vi "Test Process Multiple Parallell Processes.vi"(8 "error in (no error)":errorcluster, 11 "Rig Test In":refnum<class "Process Dev Test.lvclass">) -> (0 "error out":errorcluster, 3 "Rig Test Out":refnum<class "Process Dev Test.lvclass">)   [LabVIEW 2020, in "Process Dev Test.lvclass"]
uses:
  Process Dev Test.lvclass
  C:/Program Files (x86)/National Instruments/LabVIEW 2020/vi.lib/Astemes/LUnit/Test Case.lvclass
  source/Framework Test Suite/Mock Error Handler/Mock Error Handler.lvclass
  C:/Git/triarc-framework/source/Framework/Error Handler Interface/Error Handler Interface.lvclass
  source/Framework/Process/Process.lvclass
  source/Framework/Process/Process.lvclass/Process.ctl
  <vilib>/Astemes/LUnit/Test Case.lvclass/Test Case.ctl
  <vilib>/Astemes/LUnit/LUnit Assertion Result.lvclass/LUnit Assertion Result.ctl
  <vilib>/Astemes/LUnit/LUnit Test Case Result.lvclass/LUnit Test Case Result.ctl
  <vilib>/Astemes/LUnit/LUnit Method Result.lvclass/LUnit Method Result.ctl
  source/Framework/Process/Protected/Messaging/Enqueue Message.vi
  source/Framework/Process/Public/Lifecycle/Get Lifecycle State.vi
  source/Framework/Process/Private/SubVIs/Wait for finish.vi
  source/Framework/Process/Private/SubVIs/Set Lifecycle State.vi
  <vilib>/Astemes/LUnit/Set Assertion Type.vi
  <vilib>/Astemes/LUnit/Palette/Pass.vi
  <vilib>/Astemes/LUnit/Palette/Fail.vi
  source/Framework/Process/Private/SubVIs/Handle Debug Data.vi
  <vilib>/Utility/error.llb/Clear Errors.vi
  <vilib>/Astemes/LUnit/LUnit Write Assertion Type.vi
  <vilib>/Astemes/LUnit/Add test result.vi
  <vilib>/Astemes/LUnit/LUnit Write Passed.vi
  <vilib>/Astemes/LUnit/LUnit Write Message.vi
  <vilib>/Astemes/LUnit/LUnit Write Description.vi
  source/Framework/Logging/Log Debug.vi
  <vilib>/AdvancedString/1D String Array to Delimited String.vi
  <vilib>/Utility/High Resolution Relative Seconds.vi
  <vilib>/Astemes/LUnit/LUnit Record Assertion Result.vi
  <vilib>/Astemes/LUnit/LUnit Aggregate Assertion Results.vi
  <vilib>/Astemes/LUnit/Assertion Result/LUnit Read Status.vi
  <vilib>/Astemes/LUnit/LUnit Read Message.vi
  <vilib>/Astemes/LUnit/LUnit Read Description.vi
  <vilib>/Astemes/LUnit/Method Result/LUnit Merge Status.vi
  <vilib>/Astemes/LUnit/LUnit Concatenate result strings.vi
  <vilib>/Utility/error.llb/Error Cluster From Error Code.vi
  source/Framework/Process/Public/Read Name.vi
  <vilib>/Astemes/LUnit/LUnit Assertion Result.lvclass
  <vilib>/Astemes/LUnit/Test Case.lvclass
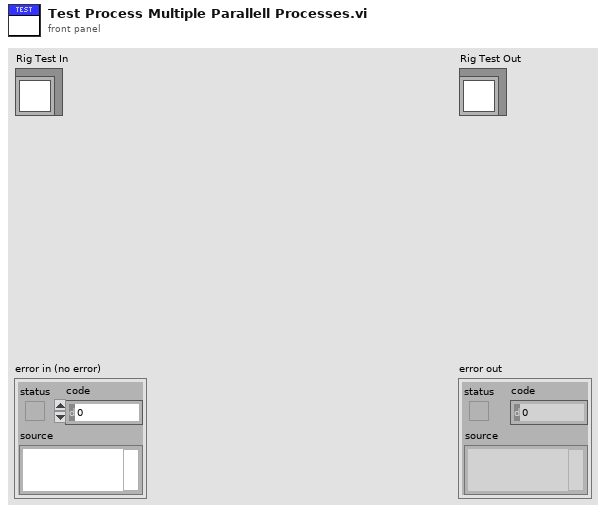
[diagram p1: front panel]
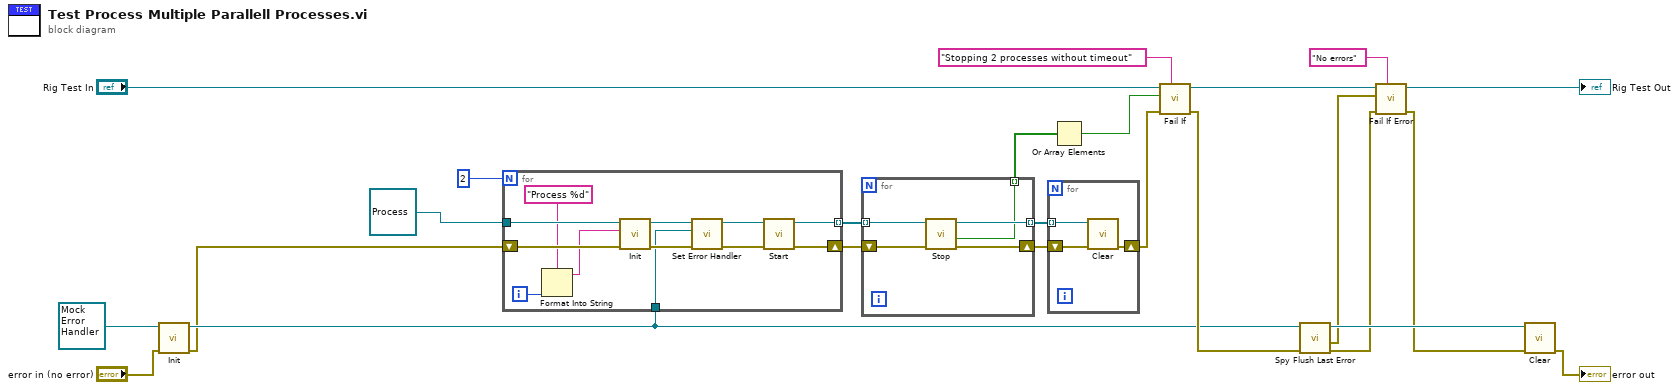
[diagram p0: block diagram]
diagram:
  n1 = call-dynamic "Init.vi"("error in (no error)"="error in (no error)", "Mock Error Handler In"=refnum<class "Mock Error Handler.lvclass"> refnum ("Mock Error Handler.lvclass")) -> ("error out"=w3:errorcluster, "Mock Error Handler Out"=w6:refnum<class "Mock Error Handler.lvclass">)  [unwired: 8 in]
  n2 = for {
    N: 2 -> [_]
    tunnel: [w36] -> w23 mode=indexing
    tunnel: refnum<class "Process.lvclass"> refnum ("Process.lvclass") -> [w33]
    shift-right: [w35] -> w22
    shift-left: w3 -> [w34]
    tunnel: w6 -> [w28]
    i -> [w26]
    n3 = Format Into String(format string="Process %d", w26) -> (resulting string=w25:string)  [unwired: 2 in, 1 out]
    n4 = call-dynamic "Init.vi"("error in (no error)"=w34, "Name"=w25, "Process In"=w33) -> ("error out"=w30:errorcluster, "Process Out"=w32:refnum<class "Process.lvclass">)  [unwired: 7 in]
    n5 = call "Set Error Handler.vi"("error in (no error)"=w30, "Error Handler"=w28, "Process In"=w32) -> ("error out"=w29:errorcluster, "Process Out"=w31:refnum<class "Process.lvclass">)  [unwired: 7 in]
    n6 = call "Start.vi"("error in (no error)"=w29, "Process In"=w31) -> ("error out"=w35:errorcluster, "Process Out"=w36:refnum<class "Process.lvclass">)  [unwired: 7 in, 1 out]
  }
  n7 = for {
    tunnel: [w37] -> w19 mode=indexing
    shift-right: [w38] -> w20
    shift-left: w22 -> [w40]
    tunnel: w23 -> [w41] mode=indexing
    tunnel: [w39] -> w21 mode=indexing
    n8 = call "Stop.vi"("error in (no error)"=w40, "Process In"=w41) -> ("error out"=w38:errorcluster, "timed out?"=w37:bool, "Process Out"=w39:refnum<class "Process.lvclass">)  [unwired: 7 in]
  }
  n9 = for {
    tunnel: w21 -> [w44] mode=indexing
    shift-right: [w42] -> w16
    shift-left: w20 -> [w43]
    n10 = call-dynamic "Clear.vi"("error in (no error)"=w43, "Process In"=w44) -> ("error out"=w42:errorcluster)  [unwired: 9 in]
  }
  n11 = Or Array Elements(Boolean array=w19) -> (logical OR=w17:bool)
  n12 = call <vilib>:"Fail If.vi"("Description"="Stopping 2 processes without timeout", "error in (no error)"=w16, "Fail?"=w17, "LUnit Test Case In"="Rig Test In") -> ("error out"=w7:errorcluster, "LUnit Test Case Out"=w24:refnum<class "Process Dev Test.lvclass">)  [unwired: 6 in]
  n13 = call "Spy Flush Last Error.vi"("error in (no error)"=w7, "Mock Error Handler In"=w6) -> ("error out"=w12:errorcluster, "Error"=w11:errorcluster, "Mock Error Handler Out"=w15:refnum<class "Mock Error Handler.lvclass">)  [unwired: 7 in]
  n14 = call <vilib>:"Fail If Error.vi"("Description"="No errors", "error in (no error)"=w12, "Assert error"=w11, "LUnit Test Case In"=w24) -> ("error out"=w9:errorcluster, "LUnit Test Case Out"=→"Rig Test Out":refnum<class "Process Dev Test.lvclass">)  [unwired: 6 in]
  n15 = call-dynamic "Clear.vi"("error in (no error)"=w9, "Mock Process In"=w15) -> ("error out"=→"error out":errorcluster)  [unwired: 9 in]
